vi "Write VisibleVerticalLines.vi"(8 "error in (no error)":errorcluster, 10 "VisibleVerticalLines":bool, 11 "Calendar in":refnum<class "Calendar.lvclass">) -> (0 "error out":errorcluster, 3 "Calendar out":refnum<class "Calendar.lvclass">)   [LabVIEW 2015, in "Calendar.lvclass"]
uses:
  Calendar.lvclass
  Calendar.lvclass/Calendar.ctl
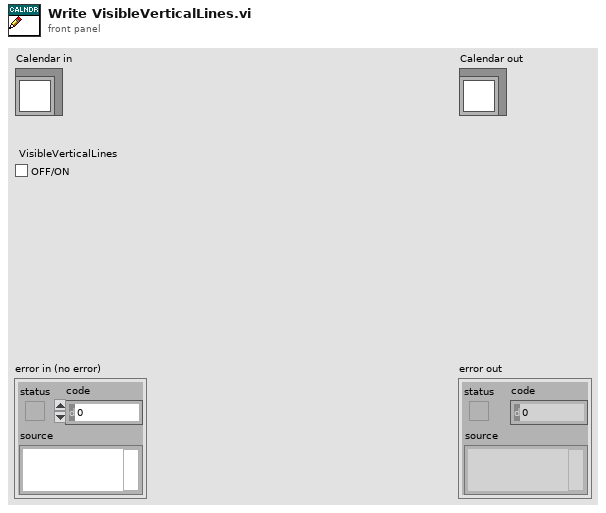
[diagram p1: front panel]
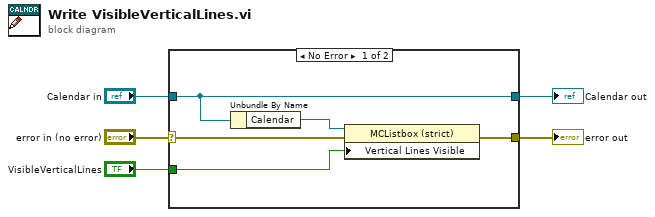
[diagram p0: block diagram]
diagram:
  n1 = case shown="No Error" "error in (no error)" {
    selector: "error in (no error)" -> [w10 w12]
    tunnel: [w8 w12] -> w4
    tunnel: [w9 w11] -> w2
    tunnel: "Calendar in" -> [w9 w11]
    tunnel: "VisibleVerticalLines" -> [w6 _]
    frame No Error {
      n2 = Unbundle By Name(w9) -> ("Calendar"=w7:refnum<vi>)
      n3 = property class="MCListbox (strict)"(reference=w7, error in=w10, "Vertical Lines Visible"=w6) -> (error out=w8:errorcluster)  [unwired: 1 out]
    }
    frame Error {
    }
  }
  "error out" <- w4
  "Calendar out" <- w2
